vi "q4 database.vi"() -> ()   [LabVIEW 2018]
panel:
  out "output array":T1(array[cluster])
  in  "marks":dbl
  in  "sub":dbl
  in  "roll":dbl
  in  "Database":T1(array[cluster])
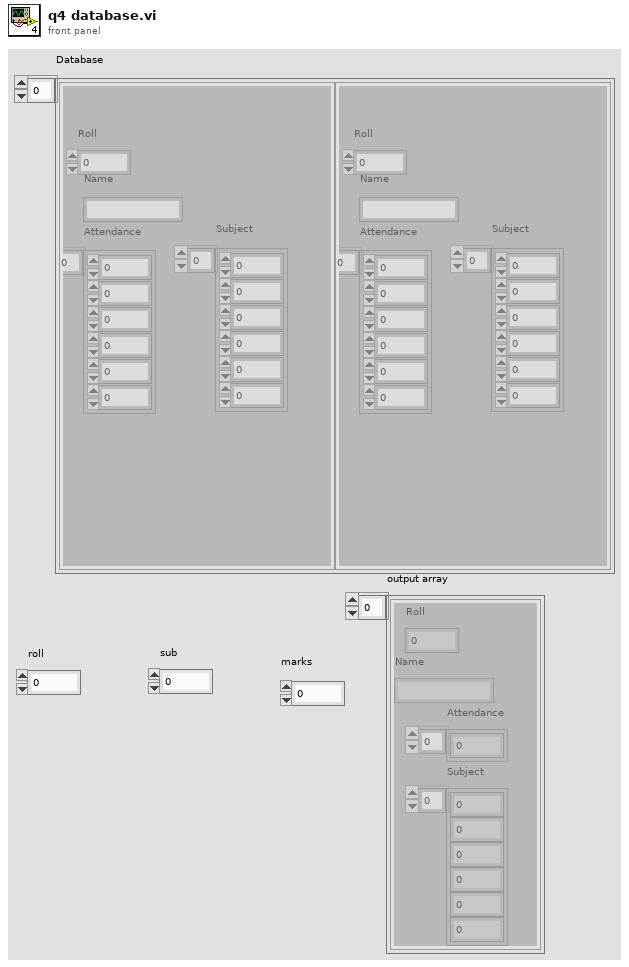
[diagram p1: front panel]
types:
  T1 = cluster{"Roll":dbl, "Name":string, "Attendance":dbl[], "Subject":dbl[]}[]
  T2 = cluster{"Roll":dbl, "Name":string, "Attendance":dbl[], "Subject":dbl[]}
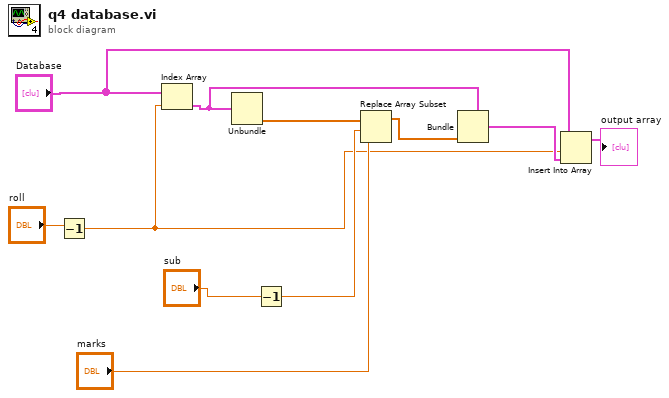
[diagram p0: block diagram]
diagram:
  n1 = Decrement(x="roll") -> (x-1=w2:dbl)
  n2 = Index Array(array="Database", index=w2) -> (element=w5:T2)
  n3 = Unbundle(w5) -> ("Subject"=w11:dbl[])  [unwired: 3 out]
  n4 = Decrement(x="sub") -> (x-1=w8:dbl)
  n5 = Replace Array Subset(array=w11, new element="marks", index=w8) -> (w6:dbl[])
  n6 = Bundle(cluster=w5, "Subject"=w6) -> (w4:T2)  [unwired: 3 in]
  n7 = Insert Into Array(array="Database", index=w2, new element=w4) -> (→"output array":T1)
